vi "WLAN - TV - RW - UTIL - StringClusterToDataType(Meas).vi"(7 "TV Paramaters(String)":T2) -> (8 "TV Parameters(DataType)":T1 {"Standard" items=["80211A/G/J/P OFDM", "80211B/G DSSS", "80211G DSSSOFDM", "80211N MIMOOFDM", "80211AC MIMOOFDM"]; "OFDM Data Rate (Mbps)" items=["6", "9", "12", "18", "24", "36", "48", "54"]; "80211n PLCP Frame Format" items=["Mixed Format", "Greenfield Format"]; "FEC Coding Type" items=["BCC", "LDPC"]; "DSSS Data Rate (Mbps)" items=["1", "2", "5.5 CCK", "5.5 PBCC", "11 CCK", "11 PBCC", "22", "33"]})   [LabVIEW 2012]
uses:
  Includes/WLAN - TV - RW - INC - TV_Parameters.ctl
  Includes/WLAN - TV - RW - INC - TV_DataType_Cluster.ctl
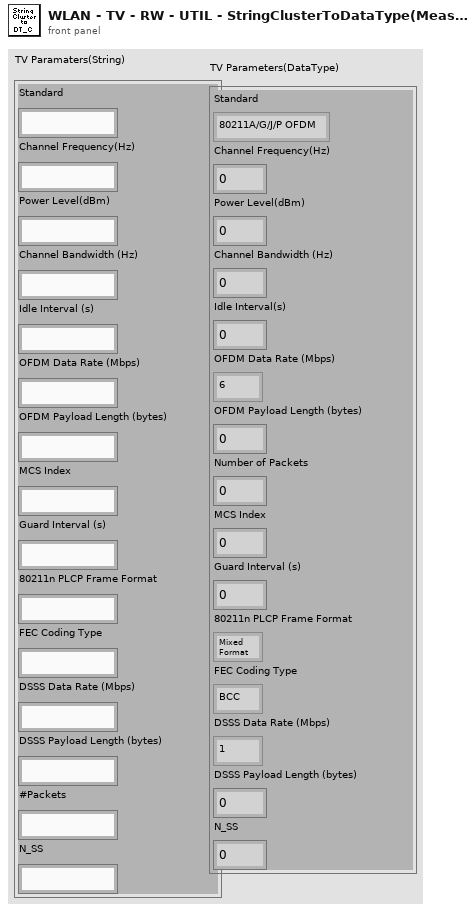
[diagram p1: front panel]
types:
  T1 = typedef "WLAN - TV - RW - INC - TV_DataType_Cluster.ctl" = cluster{"Standard":i32, "Channel Frequency(Hz)":dbl, "Power Level(dBm)":dbl, "Channel Bandwidth (Hz)":dbl, "Idle Interval(s)":dbl, "OFDM Data Rate (Mbps)":i32, "OFDM Payload Length (bytes)":i32, "Number of Packets":i32, "MCS Index":i32, "Guard Interval (s)":dbl, "80211n PLCP Frame Format":i32, "FEC Coding Type":i32, "DSSS Data Rate (Mbps)":i32, "DSSS Payload Length (bytes)":i32, "N_SS":i32}
  T2 = typedef "WLAN - TV - RW - INC - TV_Parameters.ctl" = cluster{"Standard ":string, "Channel Frequency(Hz)":string, "Power Level(dBm)":string, "Channel Bandwidth (Hz)":string, "Idle Interval (s)":string, "OFDM Data Rate (Mbps)":string, "OFDM Payload Length (bytes)":string, "MCS Index":string, "Guard Interval (s)":string, "80211n PLCP Frame Format":string, "FEC Coding Type":string, "DSSS Data Rate (Mbps)":string, "DSSS Payload Length (bytes)":string, "#Packets":string, "N_SS":string}
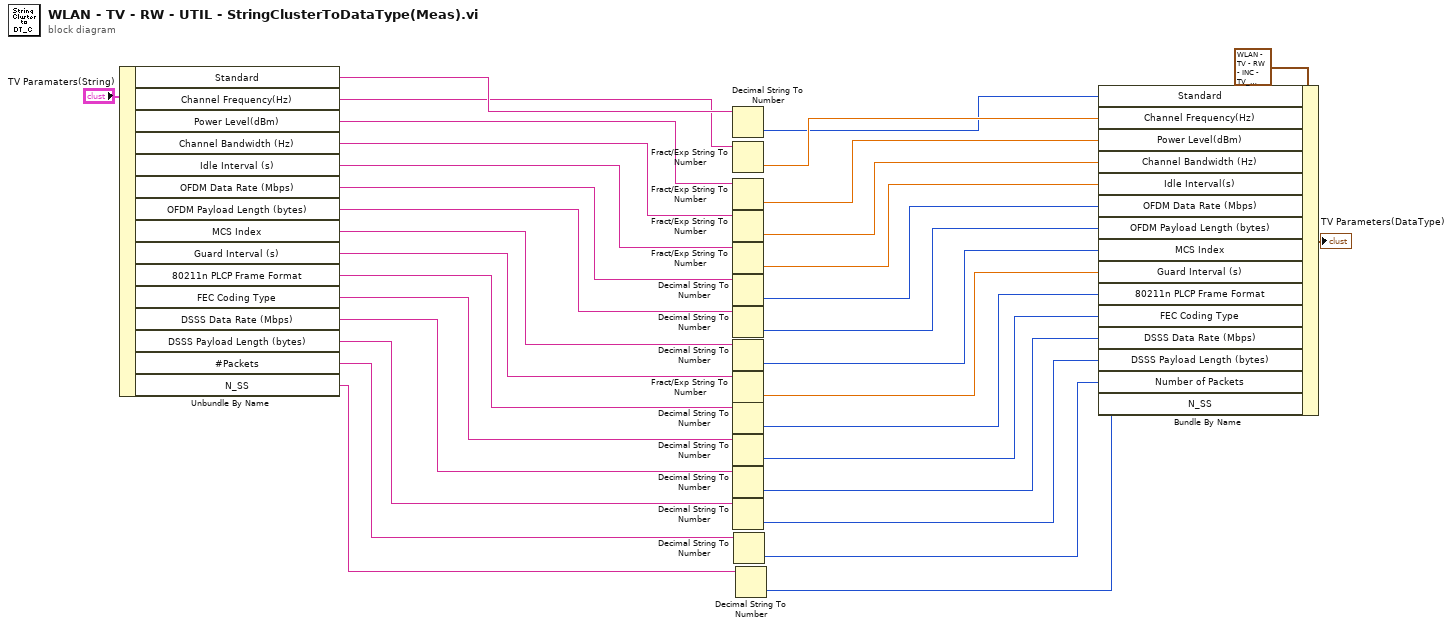
[diagram p0: block diagram]
diagram:
  n1 = Unbundle By Name("TV Paramaters(String)") -> ("Standard"=w31:string, "Channel Frequency(Hz)"=w30:string, "Power Level(dBm)"=w29:string, "Channel Bandwidth (Hz)"=w28:string, "Idle Interval (s)"=w27:string, "OFDM Data Rate (Mbps)"=w26:string, "OFDM Payload Length (bytes)"=w25:string, "MCS Index"=w24:string, "Guard Interval (s)"=w23:string, "80211n PLCP Frame Format"=w22:string, "FEC Coding Type"=w21:string, "DSSS Data Rate (Mbps)"=w20:string, "DSSS Payload Length (bytes)"=w19:string, "#Packets"=w7:string, "N_SS"=w2:string)
  n2 = Decimal String To Number(string=w31) -> (number=w9:i32)  [unwired: 2 in, 1 out]
  n3 = Fract/Exp String To Number(string=w30) -> (number=w10:dbl)  [unwired: 3 in, 1 out]
  n4 = Fract/Exp String To Number(string=w29) -> (number=w5:dbl)  [unwired: 3 in, 1 out]
  n5 = Fract/Exp String To Number(string=w28) -> (number=w11:dbl)  [unwired: 3 in, 1 out]
  n6 = Fract/Exp String To Number(string=w27) -> (number=w12:dbl)  [unwired: 3 in, 1 out]
  n7 = Decimal String To Number(string=w26) -> (number=w13:i32)  [unwired: 2 in, 1 out]
  n8 = Decimal String To Number(string=w25) -> (number=w14:i32)  [unwired: 2 in, 1 out]
  n9 = Decimal String To Number(string=w24) -> (number=w15:i32)  [unwired: 2 in, 1 out]
  n10 = Fract/Exp String To Number(string=w23) -> (number=w3:dbl)  [unwired: 3 in, 1 out]
  n11 = Decimal String To Number(string=w22) -> (number=w16:i32)  [unwired: 2 in, 1 out]
  n12 = Decimal String To Number(string=w21) -> (number=w17:i32)  [unwired: 2 in, 1 out]
  n13 = Decimal String To Number(string=w20) -> (number=w18:i32)  [unwired: 2 in, 1 out]
  n14 = Decimal String To Number(string=w19) -> (number=w8:i32)  [unwired: 2 in, 1 out]
  n15 = Decimal String To Number(string=w7) -> (number=w4:i32)  [unwired: 2 in, 1 out]
  n16 = Decimal String To Number(string=w2) -> (number=w1:i32)  [unwired: 2 in, 1 out]
  n17 = Bundle By Name(cluster=T1 {"Standard"=0, "Channel Frequency(Hz)"=0.0, "Power Level(dBm)"=0.0, "Channel Bandwidth (Hz)"=0.0, "Idle Interval(s)"=0.0, "OFDM Data Rate (Mbps)"=0, "OFDM Payload Length (bytes)"=0, "Number of Packets"=0, "MCS Index"=0, "Guard Interval (s)"=0.0, "80211n PLCP Frame Format"=0, "FEC Coding Type"=0, "DSSS Data Rate (Mbps)"=0, "DSSS Payload Length (bytes)"=0, "N_SS"=0} ("TV Parameters(DataType)"), "Standard"=w9, "Channel Frequency(Hz)"=w10, "Power Level(dBm)"=w5, "Channel Bandwidth (Hz)"=w11, "Idle Interval(s)"=w12, "OFDM Data Rate (Mbps)"=w13, "OFDM Payload Length (bytes)"=w14, "MCS Index"=w15, "Guard Interval (s)"=w3, "80211n PLCP Frame Format"=w16, "FEC Coding Type"=w17, "DSSS Data Rate (Mbps)"=w18, "DSSS Payload Length (bytes)"=w8, "Number of Packets"=w4, "N_SS"=w1) -> (→"TV Parameters(DataType)":T1)
